vi "add autopop folders.vi"(7 "private?":bool, 8 "error in (no error)":errorcluster, 10 "autopop":path[](array[path]), 11 "ProjectItem in":refnum<vi>) -> (0 "error out":errorcluster, 2 "items out":refnum<vi>[](array[refnum]), 3 "ProjectItem out":refnum<vi>)   [LabVIEW 2013]
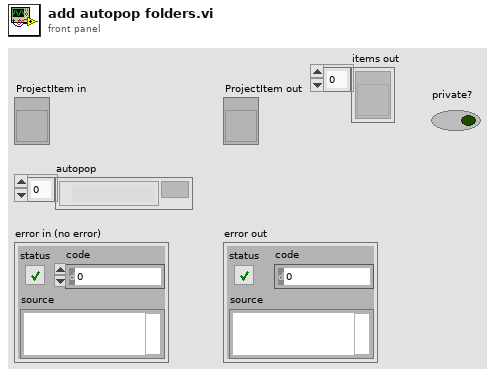
[diagram p1: front panel]
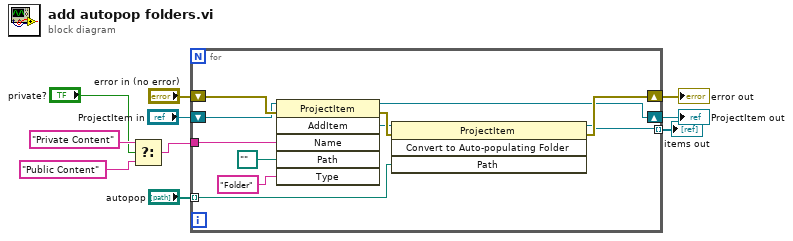
[diagram p0: block diagram]
diagram:
  n1 = Select(t="Private Content" ("folder name"), s="private?", f="Public Content" ("folder name")) -> (s? t:f=w5:string)
  n2 = for {
    shift-right: [w17] -> w10
    shift-left: "error in (no error)" -> [w21]
    tunnel: "autopop" -> [w14] mode=indexing
    shift-right: [w15] -> w9
    shift-left: "ProjectItem in" -> [w20]
    tunnel: w5 -> [w12]
    tunnel: [w11] -> w1 mode=indexing
    n3 = invoke class="ProjectItem" method="AddItem"(reference=w20, error in=w21, "Name"=w12, "Path"=path "", "Type"="Folder") -> (reference out=w15:refnum<vi>, error out=w18:errorcluster, "AddItem"=w16:refnum<vi>)  [unwired: 1 in, 3 out]
    n4 = invoke class="ProjectItem" method="Convert to Auto-populating Folder"(reference=w16, error in=w18, "Path"=w14) -> (reference out=w11:refnum<vi>, error out=w17:errorcluster)  [unwired: 1 in, 2 out]
  }
  "error out" <- w10
  "ProjectItem out" <- w9
  "items out" <- w1
